vi "niRFUtil WFM Average (DVR) (real).vi"(0 "Avg State Element DVR":T1, 5 "Data In":T2 min=0 max=127 format="%.2f", 7 "Average Mode":enum16{"Exponential", "Repeat"}(ring), 9 "Average Method":T3, 11 "error in (no error)":errorcluster, 12 "Reset?":bool=TRUE, 13 "Initialize?":bool=TRUE) -> (6 "Average Data Out":T2 min=0 max=127 format="%.2f", 8 "Average Count":i32, 15 "error out":errorcluster)   [LabVIEW 2015, in "niRFUtil.lvlib"]
doc: "(c) Copyright 2006, National Instruments, Inc. This VI may not be duplicated, sold, or distributed without written consent from National Instruments."
uses:
  niRFUtil.lvlib
  Includes/niRFUtil INC Real Array.ctl
  Includes/niRFUtil INC Average Methods.ctl
  Includes/niRFUtil INC Average State Reference (real).ctl
  Includes/niRFUtil INC Average State Data (real).ctl
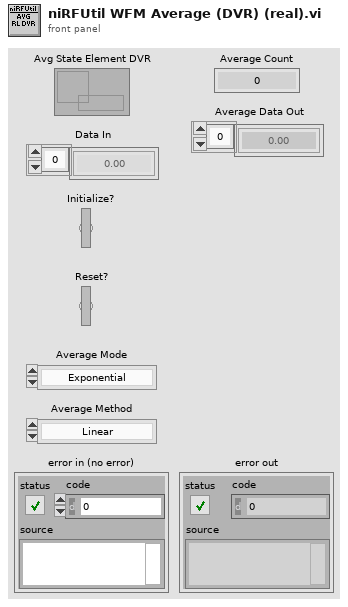
[diagram p1: front panel]
types:
  T1 = typedef "niRFUtil.lvlib/niRFUtil INC Average State Reference (real).ctl" = refnum<data-value>
  T2 = typedef "niRFUtil.lvlib/niRFUtil INC Real Array.ctl" = sgl[]
  T3 = typedef "niRFUtil.lvlib/niRFUtil INC Average Methods.ctl" = enum16{"Linear", "Log", "Root", "Max", "Min", "MinMax"}
  T4 = typedef "niRFUtil.lvlib/niRFUtil INC Average State Data (real).ctl" = cluster{"Accumulator":T2, "Count":i32}
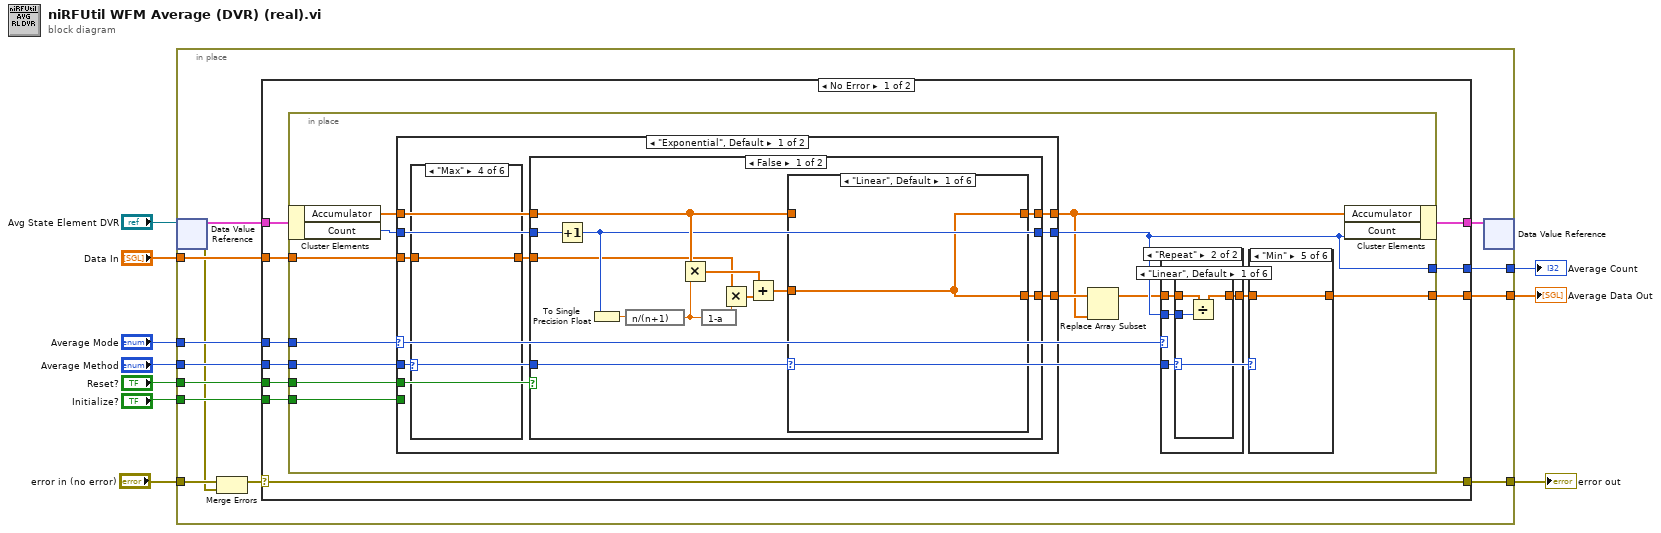
[diagram p0: block diagram]
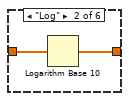
[diagram p3: hidden frame]
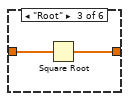
[diagram p4: hidden frame]
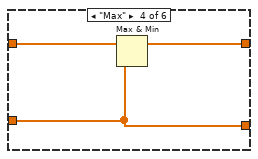
[diagram p9: hidden frame]
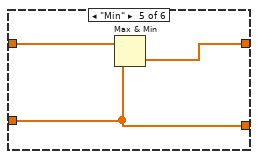
[diagram p10: hidden frame]
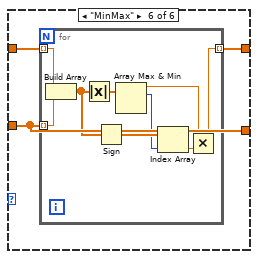
[diagram p11: hidden frame]
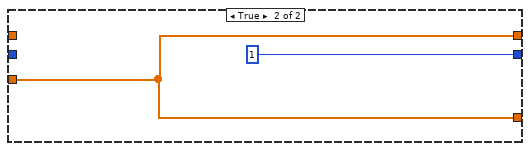
[diagram p12: hidden frame]
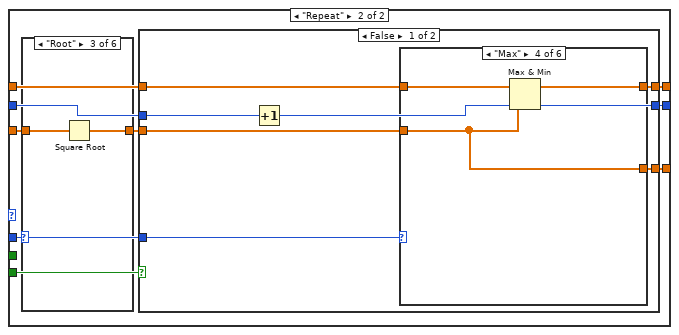
[diagram p13: hidden frame]
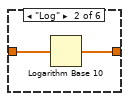
[diagram p15: hidden frame]
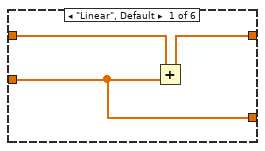
[diagram p19: hidden frame]
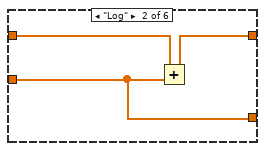
[diagram p20: hidden frame]
diagram:
  n1 = in-place {
    in-place-border: "Data In" -> [w23]
    in-place-border: "Average Mode" -> [w22]
    in-place-border: "Average Method" -> [w21]
    in-place-border: "Reset?" -> [w20]
    in-place-border: "Initialize?" -> [w19]
    in-place-border: [w18] -> w5
    in-place-border: [w15] -> w3
    in-place-border: "error in (no error)" -> [w13]
    in-place-border: [w14] -> w1
    n2 = in-place-dvr #1("Avg State Element DVR") -> (w17:T4, w12:errorcluster)
    n3 = Merge Errors(w13, w12) -> (w11:errorcluster)
    n4 = case shown="No Error" w11 {
      selector: w11 -> [w24 w178]
      tunnel: w23 -> [w33 w179]
      tunnel: w22 -> [w32 _]
      tunnel: w21 -> [w31 _]
      tunnel: w20 -> [w30 _]
      tunnel: w19 -> [w29 _]
      tunnel: [w28 w179] -> w18
      tunnel: w17 -> [w27 w180]
      tunnel: [w26 w180] -> w16
      tunnel: [w25 _] -> w15
      tunnel: [w24 w178] -> w14
      frame No Error {
        n5 = in-place {
          in-place-border: w33 -> [w46]
          in-place-border: w32 -> [w45]
          in-place-border: w31 -> [w44]
          in-place-border: w30 -> [w43]
          in-place-border: w29 -> [w42]
          in-place-border: [w38] -> w28
          in-place-border: [w37] -> w25
          n6 = in-place-cluster #2(w27) -> ("Accumulator"=w40:T2, "Count"=w39:i32)
          n7 = case shown="\"Exponential\", Default" w45 {
            tunnel: w43 -> [w52 _]
            tunnel: [w55 w108] -> w35
            tunnel: w46 -> [w50 w103]
            tunnel: [w51 w105] -> w37
            tunnel: w40 -> [w54 w107]
            tunnel: w39 -> [w53 w106]
            tunnel: w44 -> [w48 w101]
            tunnel: w42 -> [_ w104]
            tunnel: [w47 w100] -> w36
            frame "Exponential", Default {
              n8 = case shown="\"Max\"" w48 {
                tunnel: w50 -> [w56 w58 w60 w61 w62 w63]
                tunnel: [w56 w57 w59 w61 w62 w63] -> w49
                frame "Linear", Default {
                }
                frame "Log" {
                  n9 = Logarithm Base 10(1:w58) -> (0:w57:T2)
                }
                frame "Root" {
                  n10 = Square Root(x=w60) -> (sqrt(x)=w59:T2)
                }
                frame "Max" {
                }
                frame "Min" {
                }
                frame "MinMax" {
                }
              }
              n11 = case shown="False" w52 {
                tunnel: w49 -> [w65 w98]
                tunnel: [w71 w98] -> w55
                tunnel: w54 -> [w69 _]
                tunnel: w53 -> [w68 _]
                tunnel: [w67 1] -> w51
                tunnel: w48 -> [w66 _]
                tunnel: [w64 w98] -> w47
                frame False {
                  n12 = Increment(x=w68) -> (x+1=w67:i32)
                  n13 = To Single Precision Float(number=w67) -> (single precision float=w76:sgl)
                  n14 = expression code="n/(n+1)"(w76) -> (w75:sgl)
                  n15 = Multiply(x=w69, y=w75) -> (x*y=w72:T2)
                  n16 = expression code="1-a"(w75) -> (w74:sgl)
                  n17 = Multiply(x=w65, y=w74) -> (x*y=w73:T2)
                  n18 = Add(x=w72, y=w73) -> (x+y=w70:T2)
                  n19 = case shown="\"Linear\", Default" w66 {
                    tunnel: [w77 w78 w79 w81 w84 w87] -> w71
                    tunnel: w70 -> [w77 w78 w79 w80 w83 w86]
                    tunnel: w69 -> [_ _ _ w82 w85 w88]
                    tunnel: [w77 w78 w79 w80 w83 w86] -> w64
                    frame "Linear", Default {
                    }
                    frame "Log" {
                    }
                    frame "Root" {
                    }
                    frame "Max" {
                      n20 = Max & Min(x=w82, y=w80) -> (max(x,y)=w81:T2)  [unwired: 1 out]
                    }
                    frame "Min" {
                      n21 = Max & Min(x=w85, y=w83) -> (min(x,y)=w84:T2)  [unwired: 1 out]
                    }
                    frame "MinMax" {
                      n22 = for {
                        tunnel: w88 -> [w94] mode=indexing
                        tunnel: w86 -> [w93] mode=indexing
                        tunnel: [w92] -> w87 mode=indexing
                        n23 = Build Array(w94, w93) -> (w97:sgl[])
                        n24 = Absolute Value(x=w97) -> (abs(x)=w91:sgl[])
                        n25 = Sign(1:w97) -> (0:w96:sgl[])
                        n26 = Array Max & Min(array=w91) -> (max value=w90:sgl, max index (indices)=w89:i32)  [unwired: 2 out]
                        n27 = Index Array(array=w96, index=w89) -> (element=w95:sgl)
                        n28 = Multiply(x=w90, y=w95) -> (x*y=w92:sgl)
                      }
                    }
                  }
                }
                frame True {
                }
              }
            }
            frame "Repeat" {
              n29 = case shown="\"Root\"" w101 {
                tunnel: w103 -> [w109 w111 w113 w114 w115 w116]
                tunnel: [w109 w110 w112 w114 w115 w116] -> w102
                frame "Linear", Default {
                }
                frame "Log" {
                  n30 = Logarithm Base 10(1:w111) -> (0:w110:T2)
                }
                frame "Root" {
                  n31 = Square Root(x=w113) -> (sqrt(x)=w112:T2)
                }
                frame "Max" {
                }
                frame "Min" {
                }
                frame "MinMax" {
                }
              }
              n32 = case shown="False" w104 {
                tunnel: w102 -> [w118 w151]
                tunnel: [w123 w151] -> w108
                tunnel: w107 -> [w122 _]
                tunnel: w106 -> [w121 _]
                tunnel: [w120 1] -> w105
                tunnel: w101 -> [w119 _]
                tunnel: [w117 w151] -> w100
                frame False {
                  n33 = Increment(x=w121) -> (x+1=w120:i32)
                  n34 = case shown="\"Max\"" w119 {
                    tunnel: [w125 w128 w131 w134 w137 w140] -> w123
                    tunnel: w122 -> [w126 w129 w132 w135 w138 w141]
                    tunnel: w118 -> [w124 w127 w130 w133 w136 w139]
                    tunnel: [w124 w127 w130 w133 w136 w139] -> w117
                    frame "Linear", Default {
                      n35 = Add(x=w126, y=w124) -> (x+y=w125:T2)
                    }
                    frame "Log" {
                      n36 = Add(x=w129, y=w127) -> (x+y=w128:T2)
                    }
                    frame "Root" {
                      n37 = Add(x=w132, y=w130) -> (x+y=w131:T2)
                    }
                    frame "Max" {
                      n38 = Max & Min(x=w135, y=w133) -> (max(x,y)=w134:T2)  [unwired: 1 out]
                    }
                    frame "Min" {
                      n39 = Max & Min(x=w138, y=w136) -> (min(x,y)=w137:T2)  [unwired: 1 out]
                    }
                    frame "MinMax" {
                      n40 = for {
                        tunnel: w141 -> [w147] mode=indexing
                        tunnel: [w146] -> w140 mode=indexing
                        tunnel: w139 -> [w144] mode=indexing
                        n41 = Build Array(w147, w144) -> (w150:sgl[])
                        n42 = Absolute Value(x=w150) -> (abs(x)=w145:sgl[])
                        n43 = Sign(1:w150) -> (0:w149:sgl[])
                        n44 = Array Max & Min(array=w145) -> (max value=w142:sgl, max index (indices)=w143:i32)  [unwired: 2 out]
                        n45 = Index Array(array=w149, index=w143) -> (element=w148:sgl)
                        n46 = Multiply(x=w142, y=w148) -> (x*y=w146:sgl)
                      }
                    }
                  }
                }
                frame True {
                }
              }
            }
          }
          n47 = Replace Array Subset(array=w36, new element=w35) -> (w34:T2)  [unwired: 1 in]
          n48 = case shown="\"Repeat\"" w45 {
            tunnel: [w161 w163] -> w41
            tunnel: w34 -> [w161 w164]
            tunnel: w37 -> [_ w165]
            tunnel: w44 -> [_ w162]
            frame "Exponential", Default {
            }
            frame "Repeat" {
              n49 = case shown="\"Linear\", Default" w162 {
                tunnel: w165 -> [w168 w171 w174 _ _ _]
                tunnel: w164 -> [w167 w170 w173 w175 w176 w177]
                tunnel: [w166 w169 w172 w175 w176 w177] -> w163
                frame "Linear", Default {
                  n50 = Divide(x=w167, y=w168) -> (x/y=w166:T2)
                }
                frame "Log" {
                  n51 = Divide(x=w170, y=w171) -> (x/y=w169:T2)
                }
                frame "Root" {
                  n52 = Divide(x=w173, y=w174) -> (x/y=w172:T2)
                }
                frame "Max" {
                }
                frame "Min" {
                }
                frame "MinMax" {
                }
              }
            }
          }
          n53 = case shown="\"Min\"" w44 {
            tunnel: w41 -> [w153 w155 w157 w158 w159 w160]
            tunnel: [w153 w154 w156 w158 w159 w160] -> w38
            frame "Linear", Default {
            }
            frame "Log" {
              n54 = Power Of 10(x=w155) -> (10^x=w154:T2)
            }
            frame "Root" {
              n55 = Square(x=w157) -> (x^2=w156:T2)
            }
            frame "Max" {
            }
            frame "Min" {
            }
            frame "MinMax" {
            }
          }
          n56 = in-place-cluster #2("Accumulator"=w35, "Count"=w37) -> (w26:T4)
        }
      }
      frame Error {
      }
    }
    n57 = in-place-dvr #1(w16) -> ()  [unwired: 2 out]
  }
  "Average Data Out" <- w5
  "Average Count" <- w3
  "error out" <- w1
